vi "from string.vi"(8 "error in":errorcluster, 9 "data":string, 10 "version":string, 11 "Scan Engine configuration in":refnum<class "Scan Engine configuration.lvclass">) -> (0 "error out":errorcluster, 3 "Scan Engine configuration out":refnum<class "Scan Engine configuration.lvclass">)   [LabVIEW 2013, in "Scan Engine configuration.lvclass"]
doc: "Provides an interface for loading a module configuration from a file or other serialized data source. It is recommended that all children of this class store data in two sets--data required for its own initialization, and any data required for parent initialization--and that each implementation uses the <b>Call Parent Method</b> primitive to de-serialize parent information. As a result, it is expected that every module configuration class calls <b>component configuration.lvclass:From String.vi</b>."
uses:
  Scan Engine configuration.lvclass
  <vilib>/NI/Tag Bus Module Framework/channel/TBM channel.lvclass
  <vilib>/NI/Tag Bus Module Framework/module configuration/TBM module configuration.lvclass
  Scan Engine configuration.lvclass/Scan Engine configuration.ctl
  <vilib>/NI/Tag Bus Module Framework/root configuration/TBM configuration.lvclass
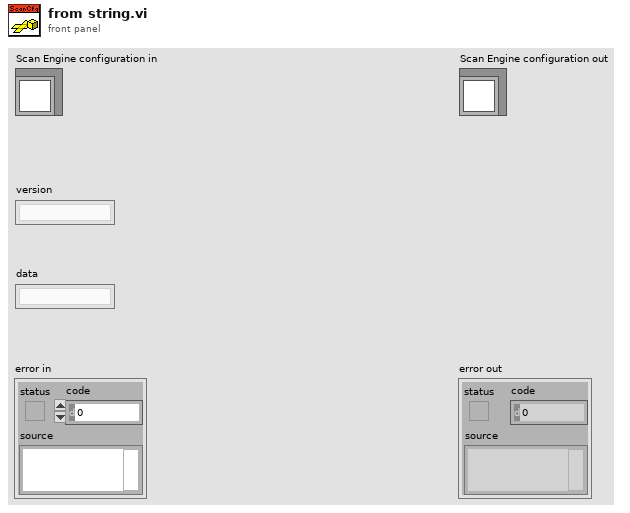
[diagram p1: front panel]
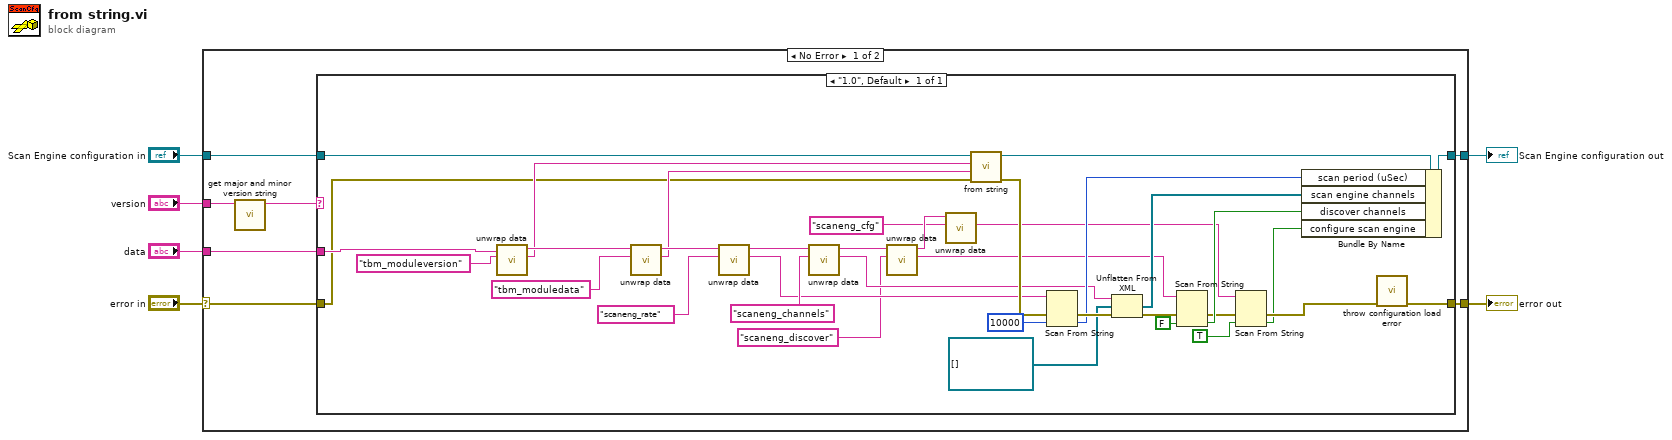
[diagram p0: block diagram]
diagram:
  n1 = case shown="No Error" "error in" {
    selector: "error in" -> [w7 w51]
    tunnel: "data" -> [w13 _]
    tunnel: "Scan Engine configuration in" -> [w12 w50]
    tunnel: [w11 w50] -> w5
    tunnel: [w10 w51] -> w4
    tunnel: "version" -> [w9 _]
    frame No Error {
      n2 = call <vilib>:"get major and minor version string.vi"("full version"=w9) -> ("major.minor version"=w8:string)  [unwired: 10 in]
      n3 = case shown="\"1.0\", Default" w8 {
        tunnel: w13 -> [w30]
        tunnel: w7 -> [w29]
        tunnel: w12 -> [w49]
        tunnel: [w45] -> w11
        tunnel: [w46] -> w10
        frame "1.0", Default {
          n4 = call <vilib>:"unwrap data.vi"("identifier"="tbm_moduleversion" ("additional identifier"), "data to unwrap"=w30) -> ("unwrapped data"=w31:string, "remaining string"=w35:string)  [unwired: 8 in]
          n5 = call <vilib>:"unwrap data.vi"("identifier"="tbm_moduledata" ("additional identifier"), "data to unwrap"=w35) -> ("unwrapped data"=w32:string, "remaining string"=w38:string)  [unwired: 8 in]
          n6 = call <vilib>:"unwrap data.vi"("identifier"="scaneng_rate" ("additional identifier"), "data to unwrap"=w38) -> ("unwrapped data"=w28:string, "remaining string"=w33:string)  [unwired: 8 in]
          n7 = call <vilib>:"unwrap data.vi"("identifier"="scaneng_channels" ("additional identifier"), "data to unwrap"=w33) -> ("unwrapped data"=w27:string, "remaining string"=w26:string)  [unwired: 8 in]
          n8 = call <vilib>:"unwrap data.vi"("identifier"="scaneng_discover" ("additional identifier"), "data to unwrap"=w26) -> ("unwrapped data"=w21:string, "remaining string"=w16:string)  [unwired: 8 in]
          n9 = call <vilib>:"unwrap data.vi"("identifier"="scaneng_cfg" ("additional identifier"), "data to unwrap"=w16) -> ("unwrapped data"=w15:string)  [unwired: 8 in, 1 out]
          n10 = call-parent "from string.vi"("error in"=w29, "data"=w32, "version"=w31, "module configuration in"=w49) -> ("error out"=w47:errorcluster, "module configuration out"=w48:refnum<class "Scan Engine configuration.lvclass">)  [unwired: 6 in]
          n11 = Scan From String(input string=w28, error in=w47, default 1=u32 10000 ("input 1")) -> (error out=w44:errorcluster, output 1=w42:u32)  [unwired: 2 in, 2 out]
          n12 = Unflatten From XML(xml string=w27, type=refnum<class "TBM channel.lvclass">[] [] ("scan engine channels"), error in (no error)=w44) -> (value=w40:refnum<class "TBM channel.lvclass">[], error out=w24:errorcluster)
          n13 = Scan From String(input string=w21, error in=w24, default 1=FALSE) -> (error out=w20:errorcluster, output 1=w22:bool)  [unwired: 2 in, 2 out]
          n14 = Scan From String(input string=w15, error in=w20, default 1=TRUE) -> (error out=w19:errorcluster, output 1=w17:bool)  [unwired: 2 in, 2 out]
          n15 = Bundle By Name(cluster=w48, "scan period (uSec)"=w42, "scan engine channels"=w40, "discover channels"=w22, "configure scan engine"=w17) -> (w45:refnum<class "Scan Engine configuration.lvclass">)
          n16 = call <vilib>:"throw configuration load error.vi"("error in"=w19) -> ("error out"=w46:errorcluster)  [unwired: 10 in]
        }
      }
    }
    frame Error {
    }
  }
  "error out" <- w4
  "Scan Engine configuration out" <- w5
